vi "VMC-3.vi"(0 "数组":u8[](array[numeric])) -> (2 "地向速度":i32, 3 "俯仰角":i16, 4 "横滚角":i16, 6 "东向速度":i32, 8 "真航向":i16, 10 "北向速度":i32, 12 "高度":i32, 13 "纬度":i32, 14 "经度":i32)   [LabVIEW 2012]
uses:
  index-i16.vi
  index-i32.vi
  XX-I16.vi
  XX-I32.vi
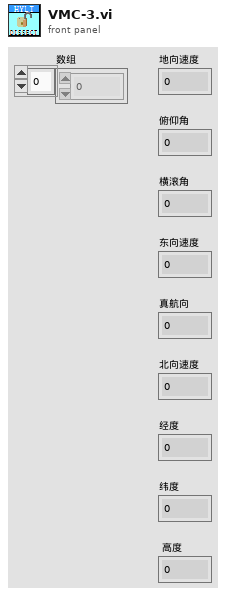
[diagram p1: front panel]
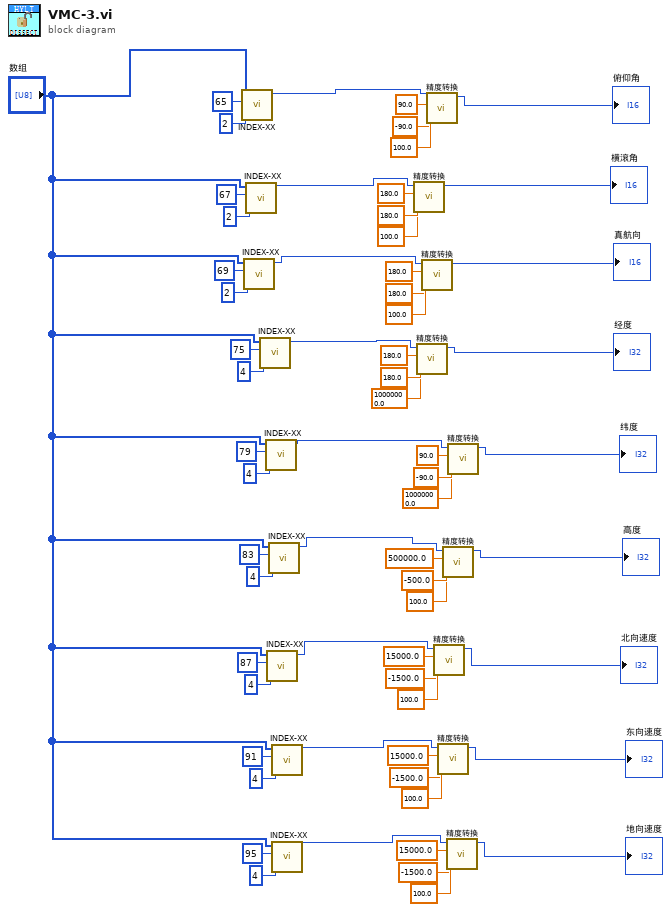
[diagram p0: block diagram]
diagram:
  n1 = call-poly "INDEX-XX.vi"("长度"=2, "索引"=65, "数组"="数组") -> ("数值输出"=w42:i16)  [unwired: 8 in]
  n2 = call-poly "INDEX-XX.vi"("长度"=2, "索引"=69, "数组"="数组") -> ("数值输出"=w32:i16)  [unwired: 8 in]
  n3 = call-poly "INDEX-XX.vi"("长度"=2, "索引"=67, "数组"="数组") -> ("数值输出"=w37:i16)  [unwired: 8 in]
  n4 = call-poly "INDEX-XX.vi"("长度"=4, "索引"=75, "数组"="数组") -> ("数值输出"=w28:i32)  [unwired: 8 in]
  n5 = call-poly "INDEX-XX.vi"("长度"=4, "索引"=79, "数组"="数组") -> ("数值输出"=w19:i32)  [unwired: 8 in]
  n6 = call-poly "INDEX-XX.vi"("长度"=4, "索引"=87, "数组"="数组") -> ("数值输出"=w12:i32)  [unwired: 8 in]
  n7 = call-poly "INDEX-XX.vi"("长度"=4, "索引"=83, "数组"="数组") -> ("数值输出"=w14:i32)  [unwired: 8 in]
  n8 = call-poly "INDEX-XX.vi"("长度"=4, "索引"=91, "数组"="数组") -> ("数值输出"=w7:i32)  [unwired: 8 in]
  n9 = call-poly "INDEX-XX.vi"("长度"=4, "索引"=95, "数组"="数组") -> ("数值输出"=w2:i32)  [unwired: 8 in]
  n10 = call-poly "精度转换.vi"("单位"=100.0, "下限"=180.0, "上限"=180.0, "数值输入"=w37) -> ("输出"=→"横滚角":i16)  [unwired: 7 in]
  n11 = call-poly "精度转换.vi"("单位"=10000000.0, "下限"=180.0, "上限"=180.0, "数值输入"=w28) -> ("输出"=→"经度":i32)  [unwired: 7 in]
  n12 = call-poly "精度转换.vi"("单位"=100.0, "下限"=180.0, "上限"=180.0, "数值输入"=w32) -> ("输出"=→"真航向":i16)  [unwired: 7 in]
  n13 = call-poly "精度转换.vi"("单位"=100.0, "下限"=-90.0, "上限"=90.0, "数值输入"=w42) -> ("输出"=→"俯仰角":i16)  [unwired: 7 in]
  n14 = call-poly "精度转换.vi"("单位"=100.0, "下限"=-1500.0, "上限"=15000.0, "数值输入"=w12) -> ("输出"=→"北向速度":i32)  [unwired: 7 in]
  n15 = call-poly "精度转换.vi"("单位"=100.0, "下限"=-1500.0, "上限"=15000.0, "数值输入"=w7) -> ("输出"=→"东向速度":i32)  [unwired: 7 in]
  n16 = call-poly "精度转换.vi"("单位"=100.0, "下限"=-500.0, "上限"=500000.0, "数值输入"=w14) -> ("输出"=→"高度":i32)  [unwired: 7 in]
  n17 = call-poly "精度转换.vi"("单位"=100.0, "下限"=-1500.0, "上限"=15000.0, "数值输入"=w2) -> ("输出"=→"地向速度":i32)  [unwired: 7 in]
  n18 = call-poly "精度转换.vi"("单位"=10000000.0, "下限"=-90.0, "上限"=90.0, "数值输入"=w19) -> ("输出"=→"纬度":i32)  [unwired: 7 in]
